vi "Test.vi"() -> ()   [LabVIEW 2020]
uses:
  TypeDefs_Utility/ENUM_NameData_String Format Select.ctl
  TypeDefs_Utility/ENUM_String_Between tolkens.ctl
panel:
  in  "tustr":T1={"Slide"=0.0, "str arry"=[[["[0,0,0]", "[0,0,1]", "[0,0,2]", "[0,0,3]"], ["[0,1,0]", "[0,1,1]", "[0,1,2]", "[0,1,3]"], ["[0,2,0]", "[0,2,1]", "[0,2,2]", "[0,2,3]"], ["[0,3,0]", "[0,3,1]", "[0,3,2]", "[0,3,3]"], ["[0,4,0]", "[0,4,1]", "[0,4,2]", "[0,4,3]"], ["[0,5,0]", "[0,5,1]", "[0,5,2]", "[0,5,3]"], ["[0,6,0]", "[0,6,1]", "[0,6,2]", "[0,6,3]"], ["[0,7,0]", "[0,7,1]", "[0,7,2]", "[0,7,3]"], ["[0,8,0]", "[0,8,1]", "[0,8,2]", "[0,8,3]"], ["[0,9,0]", "[0,9,1]", "[0,9,2]", "[0,9,3]"], ["[0,10,0]", "[0,10,1]", "[0,10,2]", "[0,10,3]"], ["[0,11,0]", "[0,11,1]", "[0,11,2]", "[0,11,3]"], ["[0,12,0]", "[0,12,1]", "[0,12,2]", "[0,12,3]"], ["[0,13,0]", "[0,13,1]", "[0,13,2]", "[0,13,3]"], ["[0,14,0]", "[0,14,1]", "[0,14,2]", "[0,14,3]"], ["[0,15,0]", "[0,15,1]", "[0,15,2]", "[0,15,3]"]], [["[1,0,0]", "[1,0,1]", "[1,0,2]", "[1,0,3]"], ["[1,1,0]", "[1,1,1]", "[1,1,2]", "[1,1,3]"], ["[1,2,0]", "[1,2,1]", "[1,2,2]", "[1,2,3]"], ["[1,3,0]", "[1,3,1]", "[1,3,2]", "[1,3,3]"], ["[1,4,0]", "[1,4,1]", "[1,4,2]", "[1,4,3]"], ["[1,5,0]", "[1,5,1]", "[1,5,2]", "[1,5,3]"], ["[1,6,0]", "[1,6,1]", "[1,6,2]", "[1,6,3]"], ["[1,7,0]", "[1,7,1]", "[1,7,2]", "[1,7,3]"], ["[1,8,0]", "[1,8,1]", "[1,8,2]", "[1,8,3]"], ["[1,9,0]", "[1,9,1]", "[1,9,2]", "[1,9,3]"], ["[1,10,0]", "[1,10,1]", "[1,10,2]", "[1,10,3]"], ["[1,11,0]", "[1,11,1]", "[1,11,2]", "[1,11,3]"], ["[1,12,0]", "[1,12,1]", "[1,12,2]", "[1,12,3]"], ["[1,13,0]", "[1,13,1]", "[1,13,2]", "[1,13,3]"], ["[1,14,0]", "[1,14,1]", "[1,14,2]", "[1,14,3]"], ["[1,15,0]", "[1,15,1]", "[1,15,2]", "[1,15,3]"]], [["[2,0,0]", "[2,0,1]", "[2,0,2]", "[2,0,3]"], ["[2,1,0]", "[2,1,1]", "[2,1,2]", "[2,1,3]"], ["[2,2,0]", "[2,2,1]", "[2,2,2]", "[2,2,3]"], ["[2,3,0]", "[2,3,1]", "[2,3,2]", "[2,3,3]"], ["[2,4,0]", "[2,4,1]", "[2,4,2]", "[2,4,3]"], ["[2,5,0]", "[2,5,1]", "[2,5,2]", "[2,5,3]"], ["[2,6,0]", "[2,6,1]", "[2,6,2]", "[2,6,3]"], ["[2,7,0]", "[2,7,1]", "[2,7,2]", "[2,7,3]"], ["[2,8,0]", "[2,8,1]", "[2,8,2]", "[2,8,3]"], ["[2,9,0]", "[2,9,1]", "[2,9,2]", "[2,9,3]"], ["[2,10,0]", "[2,10,1]", "[2,10,2]", "[2,10,3]"], ["[2,11,0]", "[2,11,1]", "[2,11,2]", "[2,11,3]"], ["[2,12,0]", "[2,12,1]", "[2,12,2]", "[2,12,3]"], ["[2,13,0]", "[2,13,1]", "[2,13,2]", "[2,13,3]"], ["[2,14,0]", "[2,14,1]", "[2,14,2]", "[2,14,3]"], ["[2,15,0]", "[2,15,1]", "[2,15,2]", "[2,15,3]"]]], "cry"=[[{"Boolean"=FALSE, "Numeric"=33.0, "bary"=[FALSE, FALSE, FALSE, FALSE, FALSE, FALSE, FALSE]}, {"Boolean"=FALSE, "Numeric"=45.0, "bary"=[FALSE, FALSE, FALSE, TRUE]}], [{"Boolean"=TRUE, "Numeric"=111.0, "bary"=[TRUE, TRUE, TRUE, TRUE, TRUE, TRUE, TRUE]}, {"Boolean"=FALSE, "Numeric"=77.0, "bary"=[TRUE, TRUE, FALSE, FALSE, FALSE, FALSE, FALSE]}], [{"Boolean"=FALSE, "Numeric"=21.0, "bary"=[TRUE, FALSE, FALSE, FALSE, FALSE, FALSE, TRUE]}, {"Boolean"=FALSE, "Numeric"=9.0, "bary"=[FALSE, FALSE, FALSE, FALSE, FALSE, TRUE, TRUE]}]], "Path"=path ""} {"Slide" scale=0.0..10.0}
  out "Values":string[](array[string])
  out "Names":string[](array[string])
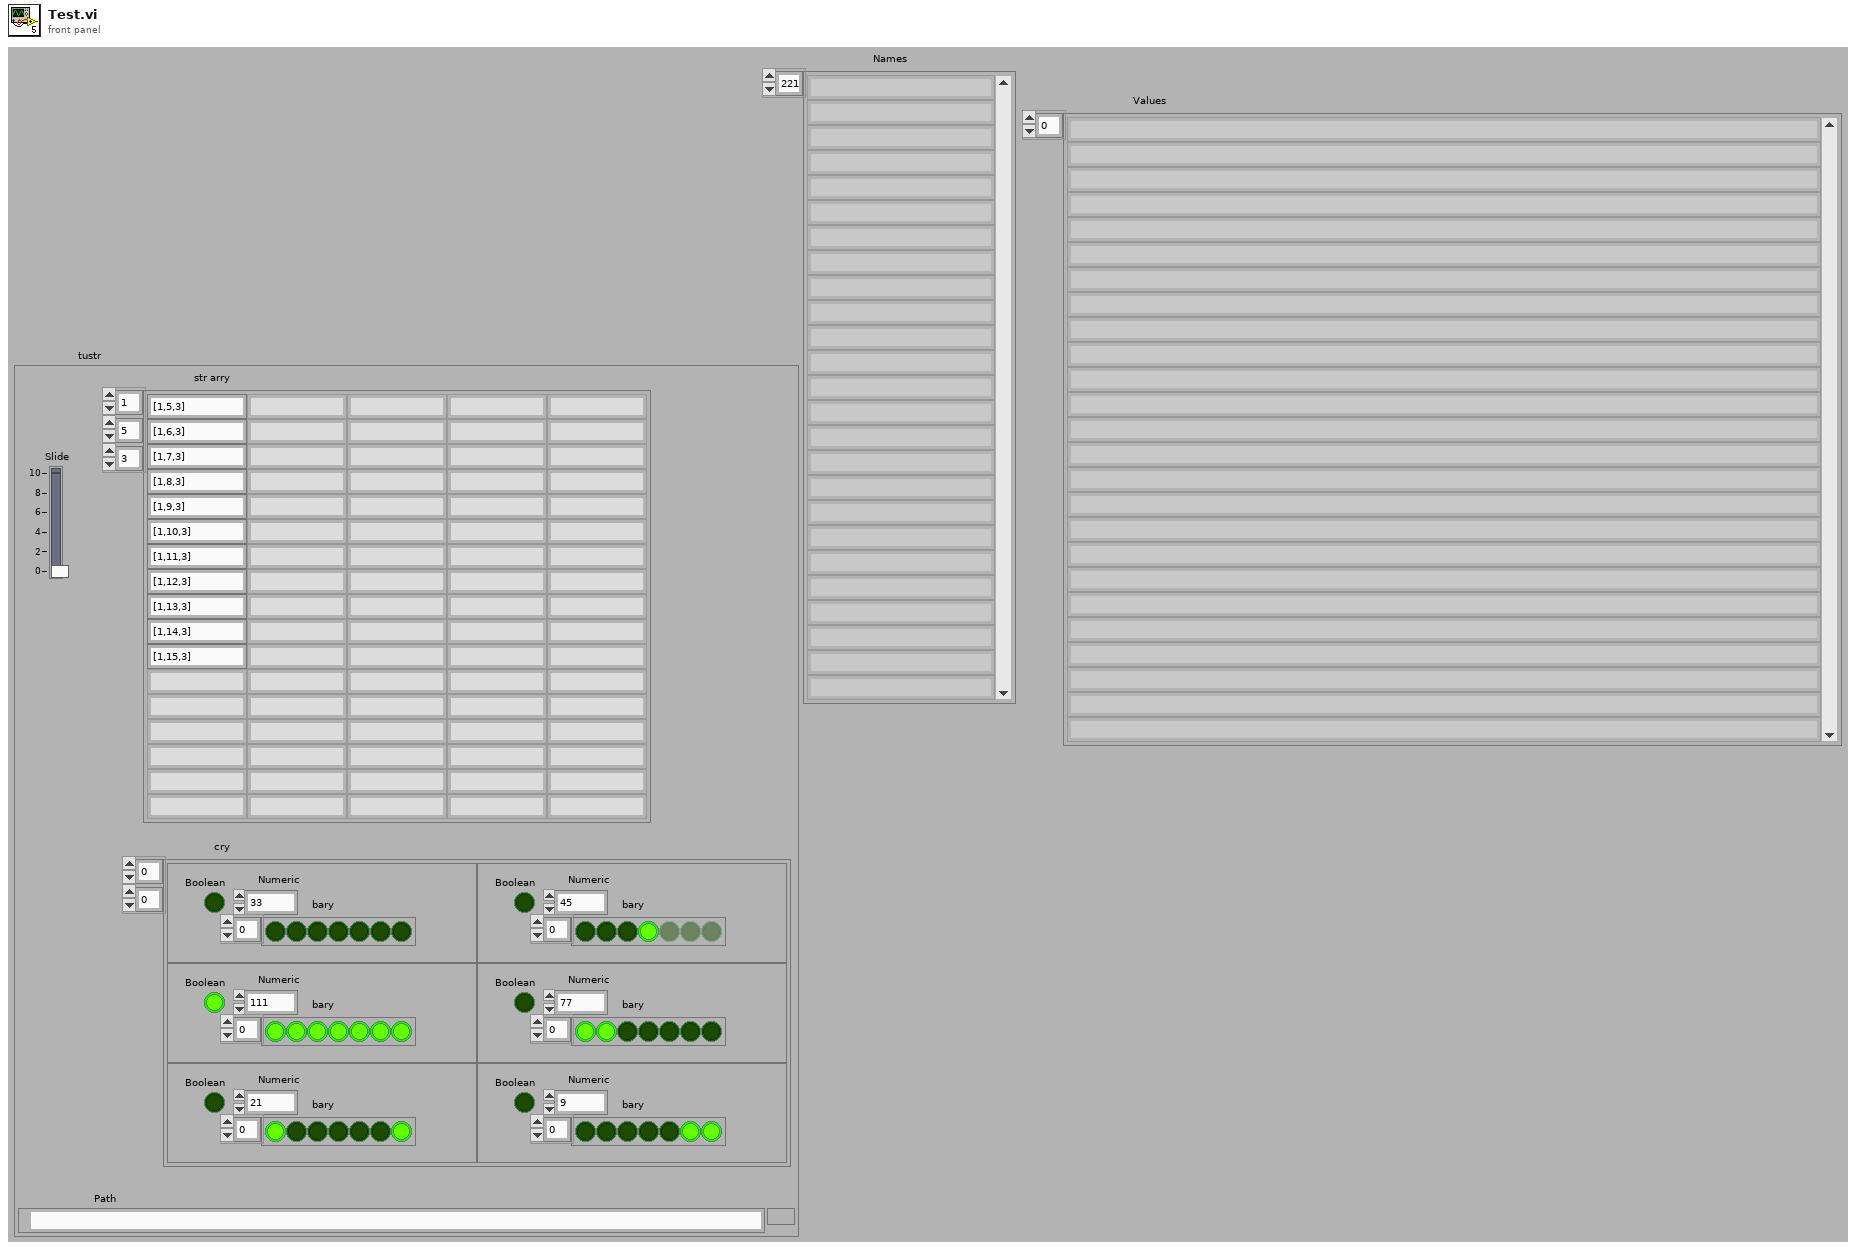
[diagram p1: front panel]
types:
  T1 = cluster{"Slide":dbl, "str arry":string[][][], "cry":cluster{"Boolean":bool, "Numeric":dbl, "bary":bool[]}[][], "Path":path}
  T2 = typedef "ENUM_NameData_String Format Select.ctl" = enum16{"Standard", "Access DB", "Custom"}
  T3 = typedef "ENUM_String_Between tolkens.ctl" = enum16{"Braces;{}", "Brackets;[]", "Parens;()", "Angles;<>", "Colens;::", "Quotes;\"\"", "Backslashes;\\\\", "None;"}
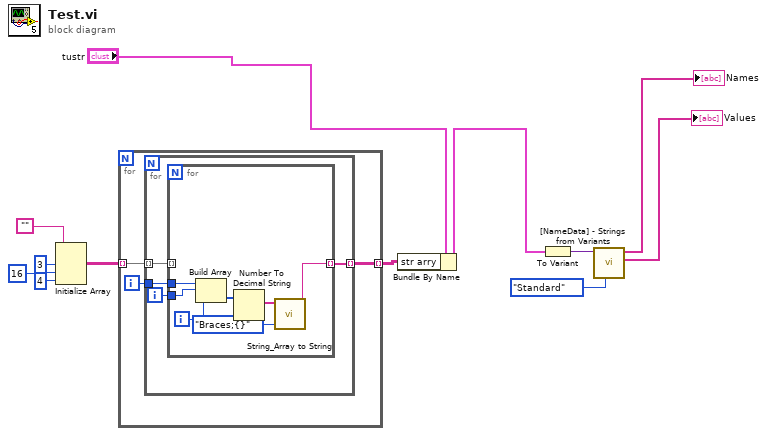
[diagram p0: block diagram]
diagram:
  n1 = Initialize Array("", 3 ("dimension size"), 16 ("dimension size"), 4 ("dimension size")) -> (w8:string[][][])
  n2 = for {
    tunnel: w8 -> [w15] mode=indexing
    tunnel: [w14] -> w4 mode=indexing
    i -> [w13]
    n3 = for {
      tunnel: w15 -> [w19] mode=indexing
      tunnel: [w18] -> w14 mode=indexing
      tunnel: w13 -> [w17]
      i -> [w16]
      n4 = for {
        tunnel: w19 -> [_] mode=indexing
        tunnel: [w20] -> w18 mode=indexing
        tunnel: w17 -> [w26]
        tunnel: w16 -> [w25]
        i -> [w24]
        n5 = Build Array(w26, w25, w24) -> (w23:i32[])
        n6 = Number To Decimal String(number=w23) -> (decimal integer string=w22:string[])  [unwired: 1 in]
        n7 = call "String_Array to String.vi"("Surround Chars"=ENUM_String_Between_tolkens."Braces;{}", "String Array"=w22) -> ("String Out"=w20:string)  [unwired: 9 in]
      }
    }
  }
  n8 = Bundle By Name(cluster="tustr", "str arry"=w4) -> (w2:T1)
  n9 = To Variant(anything=w2) -> (Variant=w1:variant)
  n10 = call "[NameData] - Strings from Variants.vi"("String Format Select"=ENUM_NameData_String_Format_Select."Standard", "Anything"=w1) -> ("Values Out"=→"Values":string[], "Names Out"=→"Names":string[])  [unwired: 5 in, 3 out]
